vi "Scripted Autonomous.vi"   [LabVIEW 2015]
uses:
  Common Code/Shooter Commands.ctl
  Common Code/Shoot Modes Enum.ctl
  Robot Global Data.vi
  Common Code/Change Detect Int.vi
types:
  T1 = typedef "Shoot Modes Enum.ctl" = enum16{"Manual", "Safe", "Auto"}
  T2 = typedef "Shooter Commands.ctl" = enum16{"Idle", "Prime Shooter", "Shoot"}
  T3 = typedef "Dashboard Control Data.ctl" = cluster{"Shooter Presets":T4, "Encoder Control":T6, "Steer PID output":cluster{"output high":dbl, "output low":dbl}, " Steer PID gains":cluster{"proportional gain (Kc)":dbl, "integral time (Ti, min)":dbl, "derivative time (Td, min)":dbl}, "Drivetrain Settings":T7, "Vision Packet":T8, "Dashboard Drivetrain Command":T9, "Info/Command Cluster":T11, "Ball Vision Packet":T12, "Intake Presets":T14, "Intake Encoder Control":T16, "Climb Presets":T17, "Goal Output Range":cluster{"output high":dbl, "output low":dbl}, "Enabled Systems":T18, "Auton Presets":T19, "Pressure M":dbl, "Pressure B":dbl, "Vision Timeout":dbl}
  T4 = typedef "Shooter Presets.ctl" = cluster{"Batter Shot":T5, "Deep Middle":T5, "Manual Shot":T5, "Left Ticks Per Rotation":dbl, "Right Ticks Per Rotation":dbl, "Low Bar Shot":T5, "Shooter RPM Tolerance":dbl, "Trigger Power":dbl, "Fire from Load Delay":i32, "Max Angle":dbl, "Min Angle":dbl, "Angle PID gains":cluster{"P":dbl, "I":dbl, "D":dbl}, "Angle Output":cluster{"output high":dbl, "output low":dbl}, "Shooter Angle Tolerance":dbl, "Vision Shoot x^2":dbl, "Vision Shoot x":dbl, "Feed Forward Max Accel":dbl, "Feed Forward Kv":dbl, "Backwards Trigger":dbl, "Shot Finish Delay (ms)":dbl, "Angle Max Current":dbl, "Angle Current Trip Time":dbl, "Intake Angle":dbl, "Vision Shoot c":dbl, "Reset?":bool, "Button Release Delay":dbl, "Angle Pot x":dbl, "Angle Pot c":dbl, "Ignore Angle?":bool, "Max RPM":dbl, "Safty Frist Angle":dbl, "Intake Danger Height":dbl, "Angle Pot B":i32, "Angle Pot M":dbl, "FF Finish RPM":dbl, "RPM PID Right":cluster{"P":dbl, "I":dbl, "D":dbl, "FF":dbl}, "RPM PID Left":cluster{"P":dbl, "I":dbl, "D":dbl, "FF":dbl}, "Backwards RPM":dbl, "Vision RPM":dbl, "Run Wheels Backward Delay":u32, "Cleat Shot":T5}
  T5 = typedef "Shot Presets.ctl" = cluster{"L":dbl, "R":dbl, "A":dbl}
  T6 = typedef "Encoder Control.ctl" = cluster{"Right Tick Constant":dbl, "Left Tick Constant":dbl, "Reset?":bool, "Y Dist":cluster{"PID gains":cluster{"proportional gain (Kc)":dbl, "integral time (Ti, min)":dbl, "derivative time (Td, min)":dbl}}, "Y Stop Thresh":dbl, "Y Stop Speed":dbl}
  T7 = typedef "Drivetrain Settings.ctl" = cluster{"Gyro Tolerance":dbl, "Throttle Ramp (ms)":dbl, "Kv":dbl, "Ka":dbl, "Feed Forward P":dbl, "Feed Forward D":dbl, "Goal Vision PID gains":cluster{"proportional gain (Kc)":dbl, "integral time (Ti, min)":dbl, "derivative time (Td, min)":dbl}, "Goal Detection Window":dbl, "Creep Rate":dbl, "Vision Throttle Threshold":dbl, "Min Turn Output":dbl, "Left Batter Angle":dbl, "Right Batter Angle":dbl}
  T8 = typedef "Goal Vision Packet.ctl" = cluster{"Distance":dbl, "Center X":dbl, "Center Y":dbl, "Found Target?":bool, "Robot Center":dbl, "Angle":dbl}
  T9 = typedef "Dashboard Drivetrain Command.ctl" = cluster{"Drivetrain Vision":T10}
  T10 = typedef "Drivetrain Vision.ctl" = cluster{"Goal Window":dbl, "Ball Window":dbl}
  T11 = typedef "Ball Tracking Command Cluster.ctl" = cluster{"Distance to Ball":dbl, "Desired Angle":dbl, "Command":enum16{"Turn to Ball", "Turn to Angle", "Get Distance"}, "Pixels from Center":dbl}
  T12 = typedef "Ball Vision Packet.ctl" = cluster{"Ball Detected?":bool, "Distance to Ball":dbl, "Desired Angle":dbl, "Pixels from Center":dbl, "Tracking mode":T13}
  T13 = typedef "Tracking Mode.ctl" = enum16{"Turn to Ball", "Turn to Angle"}
  T14 = typedef "Intake Presets.ctl" = cluster{"Intake Speed":dbl, "Outake Speed":dbl, "Low Height":dbl, "Half Height":dbl, "Full Height":dbl, "Angle Speed":dbl, "Angle Tolerance":dbl, "Encoder Scale":dbl, "Load Height":dbl, "Output Range":T15, "Rotation Power Max/Min":dbl, "MaxCurrent":dbl, "Intake Trip Time":dbl, "Idle Height":dbl, "Max Height":dbl, "Reset Encoders?":bool, "PID gains":cluster{"proportional gain (Kc)":dbl, "integral time (Ti, min)":dbl, "derivative time (Td, min)":dbl}, "Intake Stop Delay":u32, "Settle Time":dbl, "Settle Wait Time":dbl}
  T15 = typedef "Drivetrain Output Range.ctl" = cluster{"output high":dbl, "output low":dbl}
  T16 = typedef "IntakeEcoderControl.ctl" = cluster{"Arm Tick Constant":dbl, "Reset?":bool, "Y Dist":cluster{"PID gains":cluster{"proportional gain (Kc)":dbl, "integral time (Ti, min)":dbl, "derivative time (Td, min)":dbl}}, "Y Stop Thresh":dbl, "Y Stop Speed":dbl}
  T17 = typedef "Climb Presets.ctl" = cluster{"Pull Power":dbl, "Extend Power":dbl}
  T18 = typedef "Enabled Systems.ctl" = cluster{"Shoot":bool, "Intake":bool, "DT":bool, "Gyro":bool, "100ms":bool, "US":bool}
  T19 = typedef "Autonomous Presets.ctl" = cluster{"Pitch Limit":dbl, "Roll Limit":dbl, "Start Position":dbl, "Cross Position":dbl}
  T20 = typedef "Auton Command Cluster.ctl" = cluster{"Command ID":i32, "maxTime":dbl, "Y Distance":dbl, "Heading":dbl, "Throttle":dbl, "Async":dbl, "Velocity":dbl, "Acceleration":dbl, "To":dbl, "Condition":dbl, "Shot Type":dbl, "Left RPM":dbl, "Override RPM":i32, "Override Angle":i32, "Right RPM":dbl, "Angle":dbl, "Intake Mode":i32, "Intake Cmd":i32, "Intake O":i32, "Eject O":i32, "Angle O":i32, "Arm O":i32, "Intake Speed":dbl, "Eject Speed":dbl, "Arm Angle":dbl, "Arm Speed":dbl, "Intake?":i32, "Eject?":i32, "Left":dbl, "Right":dbl, "Pivot Speed":dbl, "Y Dist":dbl, "Position":dbl, "Desired Position":i32, "Shooter Mode":dbl, "Shooter Command":dbl}
  T21 = typedef "Drivetrain Status Cluster.ctl" = cluster{"Modes":T22, "Y (Throttle)":dbl, "X (Steer)":dbl, "Gyro In Range?":bool, "Distance Drive Finished?":bool, "Stop Eject Lockout":bool, "Dist Drive Status":T23, "Y Target":dbl, "Heading Target":dbl, "Vision Target Aligned?":bool, "Gear":dbl, "1st Gear Time":dbl, "2nd Gear Time":dbl, "1st Gear Shifts":dbl, "2nd Gear Shifts":dbl}
  T22 = typedef "Drivetrain Modes.ctl" = enum16{"Tank", "Climb", "Manual", "Goal Vision Targeting", "PID Distance Drive", "Hybrid", "Gyro Steer"}
  T23 = typedef "Dist Drive Status.ctl" = cluster{"Y In Range":bool, "X In Range":bool, "Gyro In Range":bool, "Y Dist":dbl, "X Dist":dbl, "Gyro":dbl}
  T24 = typedef "Drivetrain Commands.ctl" = cluster{"Y Power":dbl, "Turn Power":dbl, "2nd Gear?":bool, "Modes":T22, "Heading Target":dbl, "X Max Speed":dbl, "Y Max Speed":dbl, "X Min Speed":dbl, "Y Min Speed":dbl, "Y Target":dbl, "Max Accel":dbl, "Max Velocity":dbl, "Y Power 2":dbl, "Pivot Speed":dbl}
  T25 = typedef "Shooter Command Cluster.ctl" = cluster{"Command":T2, "Mode":T1, "Shot Type":T26, "Override Trigger Sensor":bool, "Override Angle?":bool, "Hide From Death":bool}
  T26 = typedef "Shot Type.ctl" = enum16{"Batter Shot", "Corner Shot", "Cleat Shot", "Vision Shot", "Deep Middle Shot"}
  T27 = typedef "Manual Shoot.ctl" = cluster{"Spin Wheels":bool, "Fire":bool, "Angle":dbl, "Angle Power":dbl, "Use Manual Angle":bool, "Override RPM":bool, "Left RPM":dbl, "Right RPM":dbl, "Secure Ball?":bool}
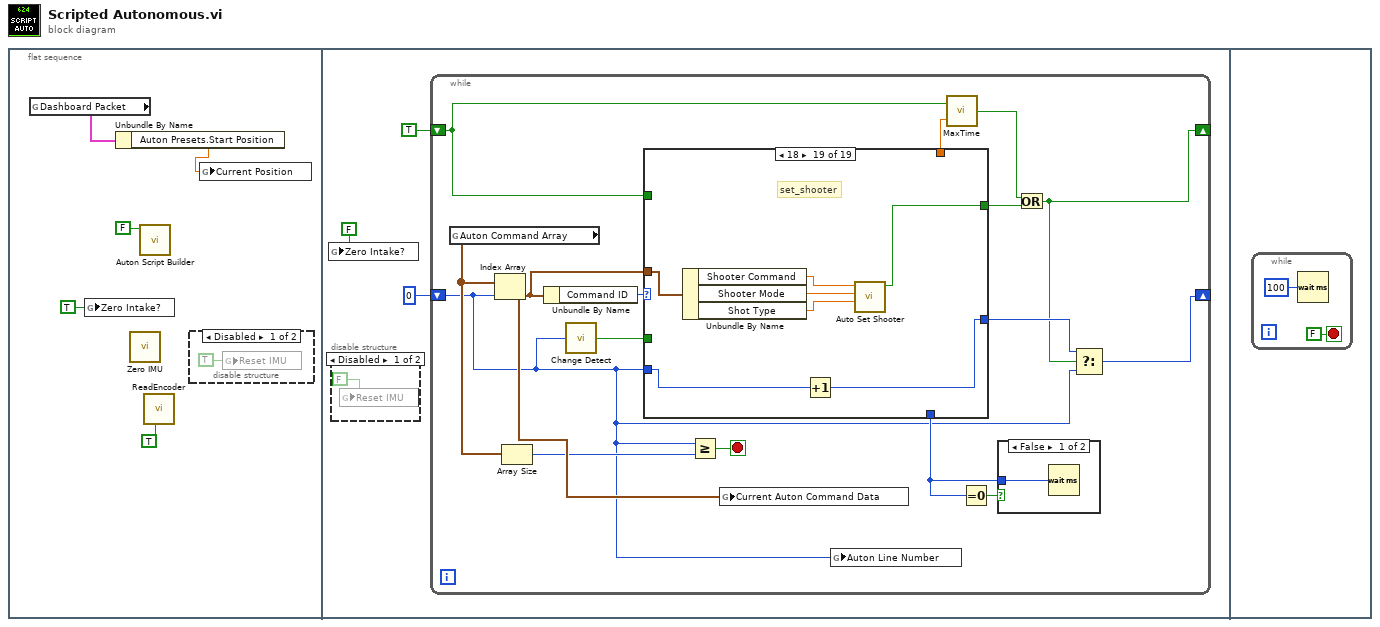
[diagram p0: block diagram]
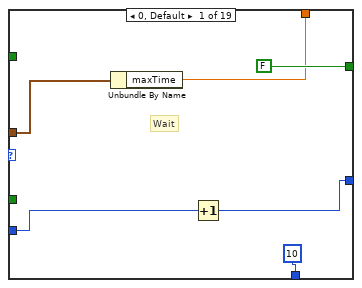
[diagram p5: hidden frame]
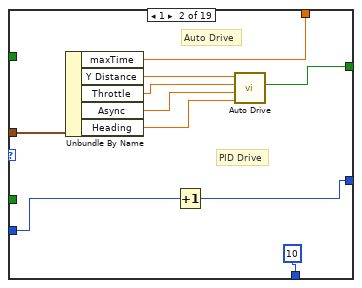
[diagram p6: hidden frame]
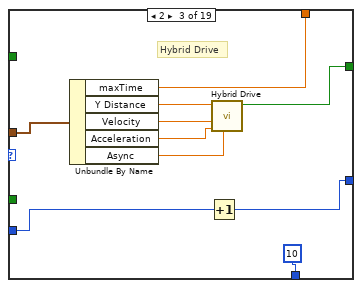
[diagram p7: hidden frame]
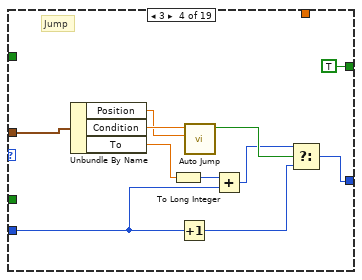
[diagram p8: hidden frame]
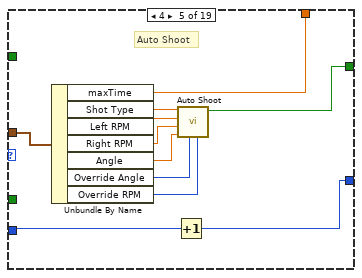
[diagram p9: hidden frame]
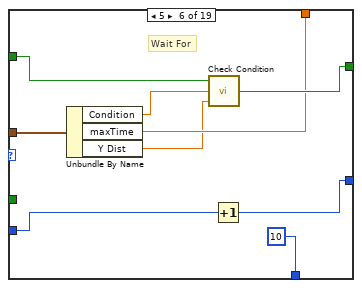
[diagram p10: hidden frame]
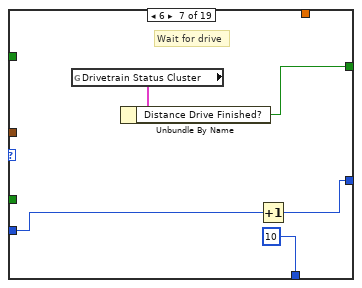
[diagram p11: hidden frame]
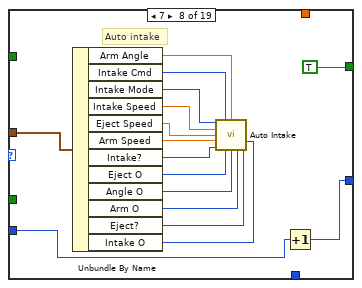
[diagram p12: hidden frame]
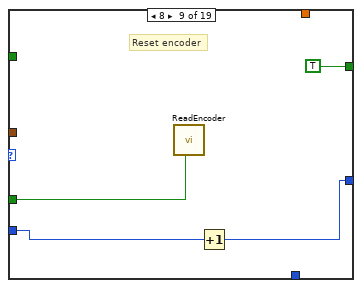
[diagram p13: hidden frame]
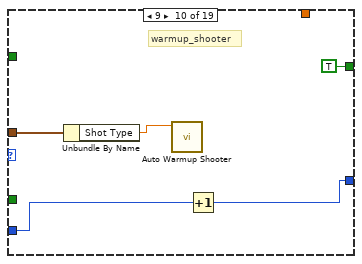
[diagram p14: hidden frame]
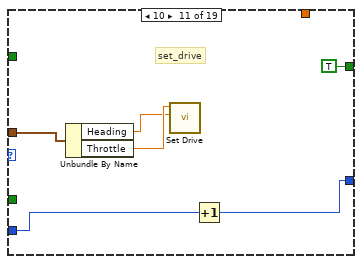
[diagram p15: hidden frame]
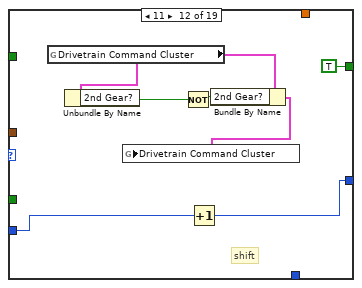
[diagram p16: hidden frame]
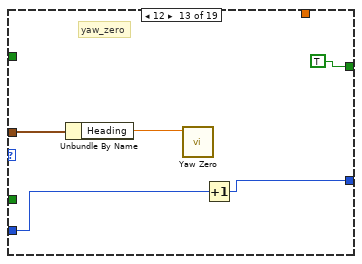
[diagram p17: hidden frame]
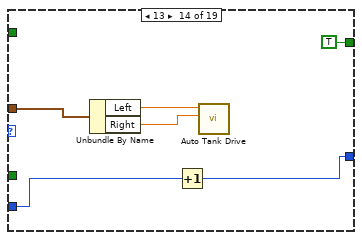
[diagram p18: hidden frame]
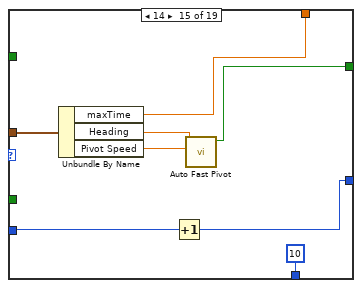
[diagram p19: hidden frame]
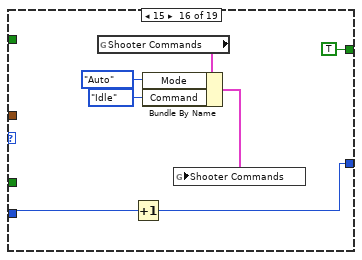
[diagram p20: hidden frame]
diagram:
  n1 = flat-sequence {
    frame #0 {
      n2 = global read "Robot Global Data.vi" "Dashboard Packet"() -> (w2:T3)
      n3 = global write "Robot Global Data.vi" "Zero Intake?"(TRUE ("Zero Intake?")) -> ()
      n4 = Unbundle By Name(w2) -> ("Auton Presets.Start Position"=w1:dbl)
      n5 = call "Zero IMU.vi"() -> ()  [unwired: 12 in]
      n6 = call "Auton Script Builder.vi"("Export?"=FALSE) -> ()  [unwired: 11 in]
      n7 = call "ReadEncoder.vi"("Reset?"=TRUE) -> ()  [unwired: 10 in, 1 out]
      n8 = disable-structure shown="Disabled" {
        frame Disabled {
          n9 = global write "Robot Global Data.vi" "Reset IMU"(TRUE ("Reset IMU")) -> ()
        }
        frame Enabled {
        }
      }
      n10 = global write "Robot Global Data.vi" "Current Position"(w1) -> ()
    }
    frame #1 {
      n11 = global write "Robot Global Data.vi" "Zero Intake?"(FALSE ("Zero Intake?")) -> ()
      n12 = disable-structure shown="Disabled" {
        frame Disabled {
          n13 = global write "Robot Global Data.vi" "Reset IMU"(FALSE ("Reset IMU")) -> ()
        }
        frame Enabled {
        }
      }
      n14 = while {
        shift-right: [w20] -> _
        shift-left: 0 -> [w11]
        shift-right: [w17] -> _
        shift-left: TRUE -> [w14]
        stop <- w21 stop-if-true
        n15 = global read "Robot Global Data.vi" "Auton Command Array"() -> (w23:T20[])
        n16 = Index Array(array=w23, index=w11) -> (element=w26:T20)
        n17 = Array Size(array=w23) -> (size(s)=w22:i32)
        n18 = Unbundle By Name(w26) -> ("Command ID"=w25:i32)
        n19 = call-poly "Change Detect.vi"("In"=w11) -> ("Changed?"=w24:bool)
        n20 = case shown="18" w25 {
          tunnel: w11 -> [w31 w36 w46 w59 w66 w78 w88 w91 w107 w112 w118 w122 w131 w135 w141 w148 w156 _ w175]
          tunnel: w24 -> [_ _ _ _ _ _ _ _ w109 _ _ _ _ _ _ _ _ _ _]
          tunnel: w14 -> [_ _ _ _ _ w84 _ _ _ _ _ _ _ _ _ _ _ _ _]
          tunnel: [w32 w35 w45 w55 w65 w76 w89 w90 w106 w111 w117 w121 w130 w134 w140 w147 w155 _ w174] -> w19
          tunnel: [FALSE w37 w49 TRUE ("Distance Drive Finished?") w67 w83 w87 TRUE TRUE ("Distance Drive Finished?") TRUE ("Distance Drive Finished?") TRUE ("Distance Drive Finished?") TRUE ("Distance Drive Finished?") TRUE TRUE ("Distance Drive Finished?") w143 TRUE ("Done?") TRUE ("Done?") w165 w169] -> w18
          tunnel: [w29 w42 w47 _ w68 w81 _ _ _ _ _ _ _ _ w142 _ _ _ _] -> w15
          tunnel: w26 -> [w30 w43 w53 w63 w75 w79 _ w104 _ w114 w120 _ w129 w138 w146 _ _ w168 w173]
          tunnel: [10 10 10 _ _ 10 10 _ _ _ _ _ _ _ 10 _ _ _ _] -> w13
          frame 0, Default {
            # "Wait"
            n21 = Unbundle By Name(w30) -> ("maxTime"=w29:dbl)
            n22 = Increment(x=w31) -> (x+1=w32:i32)
          }
          frame 1 {
            # "Auto Drive"
            # "PID Drive"
            n23 = Unbundle By Name(w43) -> ("maxTime"=w42:dbl, "Y Distance"=w41:dbl, "Throttle"=w40:dbl, "Async"=w39:dbl, "Heading"=w38:dbl)
            n24 = Increment(x=w36) -> (x+1=w35:i32)
            n25 = call "Auto Drive.vi"("heading"=w38, "async"=w39, "speed"=w40, "y"=w41) -> ("isFinished?"=w37:bool)  [unwired: 7 in]
          }
          frame 2 {
            # "Hybrid Drive"
            n26 = Unbundle By Name(w53) -> ("maxTime"=w47:dbl, "Y Distance"=w52:dbl, "Velocity"=w51:dbl, "Acceleration"=w50:dbl, "Async"=w48:dbl)
            n27 = Increment(x=w46) -> (x+1=w45:i32)
            n28 = call "Hybrid Drive.vi"("Async?"=w48, "Max Accel"=w50, "Max Velocity"=w51, "Distance"=w52) -> ("Finished?"=w49:bool)  [unwired: 7 in]
          }
          frame 3 {
            # "Jump"
            n29 = Unbundle By Name(w63) -> ("Position"=w54:dbl, "Condition"=w62:dbl, "To"=w57:dbl)
            n30 = To Long Integer(number=w57) -> (32bit integer=w58:i32)
            n31 = Increment(x=w59) -> (x+1=w60:i32)
            n32 = call "Auto Jump.vi"("Position"=w54, "Condition"=w62) -> ("Jump?"=w61:bool)  [unwired: 9 in]
            n33 = Add(x=w58, y=w59) -> (x+y=w56:i32)
            n34 = Select(t=w56, s=w61, f=w60) -> (s? t:f=w55:i32)
          }
          frame 4 {
            # "Auto Shoot"
            n35 = Unbundle By Name(w75) -> ("maxTime"=w68:dbl, "Shot Type"=w74:dbl, "Left RPM"=w73:dbl, "Right RPM"=w72:dbl, "Angle"=w71:dbl, "Override Angle"=w70:i32, "Override RPM"=w69:i32)
            n36 = Increment(x=w66) -> (x+1=w65:i32)
            n37 = call "Auto Shoot.vi"("RPM Override?"=w69, "Angle Override?"=w70, "Angle"=w71, "Right RPM"=w72, "Left RPM"=w73, "Shot Type"=w74) -> ("Finished?"=w67:bool)  [unwired: 5 in]
          }
          frame 5 {
            # "Wait For"
            n38 = Unbundle By Name(w79) -> ("Condition"=w82:dbl, "maxTime"=w81:dbl, "Y Dist"=w80:dbl)
            n39 = call "Check Condition.vi"("Distance"=w80, "Condition"=w82, "Reset"=w84) -> ("Done"=w83:bool)
            n40 = Increment(x=w78) -> (x+1=w76:i32)
          }
          frame 6 {
            # "Wait for drive"
            n41 = global read "Robot Global Data.vi" "Drivetrain Status Cluster"() -> (w86:T21)
            n42 = Unbundle By Name(w86) -> ("Distance Drive Finished?"=w87:bool)
            n43 = Increment(x=w88) -> (x+1=w89:i32)
          }
          frame 7 {
            # "Auto intake"
            n44 = Unbundle By Name(w104) -> ("Arm Angle"=w103:dbl, "Intake Cmd"=w102:i32, "Intake Mode"=w101:i32, "Intake Speed"=w100:dbl, "Eject Speed"=w99:dbl, "Arm Speed"=w98:dbl, "Intake?"=w97:i32, "Eject O"=w96:i32, "Angle O"=w95:i32, "Arm O"=w94:i32, "Eject?"=w93:i32, "Intake O"=w92:i32)
            n45 = call "Auto Intake.vi"("Intake Mode ID"=w101, "Intake Command ID"=w102, "Arm Angle"=w103, "Intake Override Speed"=w100, "Eject Override Speed"=w99, "Arm Speed"=w98, "Override Intake?"=w92, "Intake?"=w97, "Override Eject?"=w96, "Override Angle?"=w95, "Override Arm?"=w94, "Eject?"=w93) -> ()  [unwired: 4 in]
            n46 = Increment(x=w91) -> (x+1=w90:i32)
          }
          frame 8 {
            # "Reset encoder"
            n47 = call "ReadEncoder.vi"("Reset?"=w109) -> ()  [unwired: 10 in, 1 out]
            n48 = Increment(x=w107) -> (x+1=w106:i32)
          }
          frame 9 {
            # "warmup_shooter"
            n49 = Unbundle By Name(w114) -> ("Shot Type"=w113:dbl)
            n50 = call "Auto Warmup Shooter.vi"("Shot Type"=w113) -> ()  [unwired: 11 in]
            n51 = Increment(x=w112) -> (x+1=w111:i32)
          }
          frame 10 {
            # "set_drive"
            n52 = Unbundle By Name(w120) -> ("Heading"=w115:dbl, "Throttle"=w116:dbl)
            n53 = call "Set Drive.vi"("Heading Target"=w115, "Y Power"=w116) -> ()  [unwired: 10 in]
            n54 = Increment(x=w118) -> (x+1=w117:i32)
          }
          frame 11 {
            # "shift"
            n55 = global read "Robot Global Data.vi" "Drivetrain Command Cluster"() -> (w127:T24)
            n56 = Unbundle By Name(w127) -> ("2nd Gear?"=w126:bool)
            n57 = Not(x=w126) -> (.not. x?=w125:bool)
            n58 = Increment(x=w122) -> (x+1=w121:i32)
            n59 = Bundle By Name(cluster=w127, "2nd Gear?"=w125) -> (w124:T24)
            n60 = global write "Robot Global Data.vi" "Drivetrain Command Cluster"(w124) -> ()
          }
          frame 12 {
            # "yaw_zero"
            n61 = Unbundle By Name(w129) -> ("Heading"=w128:dbl)
            n62 = call "Yaw Zero.vi"("Angle"=w128) -> ()  [unwired: 11 in]
            n63 = Increment(x=w131) -> (x+1=w130:i32)
          }
          frame 13 {
            n64 = Unbundle By Name(w138) -> ("Left"=w137:dbl, "Right"=w136:dbl)
            n65 = Increment(x=w135) -> (x+1=w134:i32)
            n66 = call "Auto Tank Drive.vi"("Right"=w136, "Left"=w137) -> ()  [unwired: 10 in]
          }
          frame 14 {
            n67 = Unbundle By Name(w146) -> ("maxTime"=w142:dbl, "Heading"=w144:dbl, "Pivot Speed"=w145:dbl)
            n68 = Increment(x=w141) -> (x+1=w140:i32)
            n69 = call "Auto Fast Pivot.vi"("Pivot Speed"=w145, "Heading"=w144) -> ("Done?"=w143:bool)  [unwired: 9 in]
          }
          frame 15 {
            n70 = global read "Robot Global Data.vi" "Shooter Commands"() -> (w153:T25)
            n71 = Increment(x=w148) -> (x+1=w147:i32)
            n72 = Bundle By Name(cluster=w153, "Mode"=Shoot_Modes_Enum."Auto", "Command"=Shooter_Commands."Idle") -> (w150:T25)
            n73 = global write "Robot Global Data.vi" "Shooter Commands"(w150) -> ()
          }
          frame 16 {
            n74 = global read "Robot Global Data.vi" "Dashboard Packet"() -> (w158:T3)
            n75 = Unbundle By Name(w158) -> ("Shooter Presets.Safty Frist Angle"=w157:dbl)
            n76 = global read "Robot Global Data.vi" "Shooter Commands"() -> (w164:T25)
            n77 = global read "Robot Global Data.vi" "Manual Shoot"() -> (w161:T27)
            n78 = Bundle By Name(cluster=w164, "Mode"=Shoot_Modes_Enum."Manual") -> (w162:T25)
            n79 = global write "Robot Global Data.vi" "Shooter Commands"(w162) -> ()
            n80 = Bundle By Name(cluster=w161, "Use Manual Angle"=TRUE, "Angle"=w157) -> (w160:T27)
            n81 = global write "Robot Global Data.vi" "Manual Shoot"(w160) -> ()
            n82 = Increment(x=w156) -> (x+1=w155:i32)
          }
          frame 17 {
            n83 = Unbundle By Name(w168) -> ("Desired Position"=w166:i32)
            n84 = global read "Robot Global Data.vi" "Current Position"() -> (w167:dbl)
            n85 = call "Auto Position Drive.vi"("Desired Position"=w166, "Current Position"=w167) -> ("Finished?"=w165:bool)  [unwired: 9 in]
          }
          frame 18 {
            # "set_shooter"
            n86 = Unbundle By Name(w173) -> ("Shooter Command"=w172:dbl, "Shooter Mode"=w171:dbl, "Shot Type"=w170:dbl)
            n87 = Increment(x=w175) -> (x+1=w174:i32)
            n88 = call "Auto Set Shooter.vi"("Shot Type"=w170, "Mode"=w171, "Command"=w172) -> ("Finished?"=w169:bool)  [unwired: 8 in]
          }
        }
        n89 = Greater Or Equal?(x=w11, y=w22) -> (x >= y?=w21:bool)
        n90 = global write "Robot Global Data.vi" "Current Auton Command Data"(w26) -> ()
        n91 = global write "Robot Global Data.vi" "Auton Line Number"(w11) -> ()
        n92 = call "MaxTime.vi"("MaxTime"=w15, "Reset?"=w14) -> ("Finished?"=w16:bool)
        n93 = Equal To 0?(x=w13) -> (x = 0?=w12:bool)
        n94 = case shown="False" w12 {
          tunnel: w13 -> [w27 _]
          frame False {
            n95 = Wait (ms)(milliseconds to wait=w27) -> ()  [unwired: 1 out]
          }
          frame True {
          }
        }
        n96 = Or(x=w16, y=w18) -> (x .or. y?=w17:bool)
        n97 = Select(t=w19, s=w17, f=w11) -> (s? t:f=w20:i32)
      }
    }
    frame #2 {
      n98 = while {
        stop <- FALSE stop-if-true
        n99 = Wait (ms)(milliseconds to wait=u32 100) -> ()  [unwired: 1 out]
      }
    }
  }
